vi "Add After Undo.vi"(11 "Test Case In":refnum<class "Undo Redo Core.lvclass">) -> (0 "error out":errorcluster, 3 "Test Case Out":refnum<class "Undo Redo Core.lvclass">)   [LabVIEW 2021, in "Undo Redo Core.lvclass"]
uses:
  Undo Redo Core.lvclass
  <resource>/plugins/NIIconEditor/Controls/Undo Redo Action.ctl
  4993e8ee-a06a-463a-9684-69129f64d5ce.vi
panel:
  out "Additional Add Variables":T1
  out "Undo Variables":T2(array[cluster])
  out "Current State Variables":T1
  out "Add Variables":T2(array[cluster])
  out "Undo State Output":string[](array[string])
  out "Current State":string
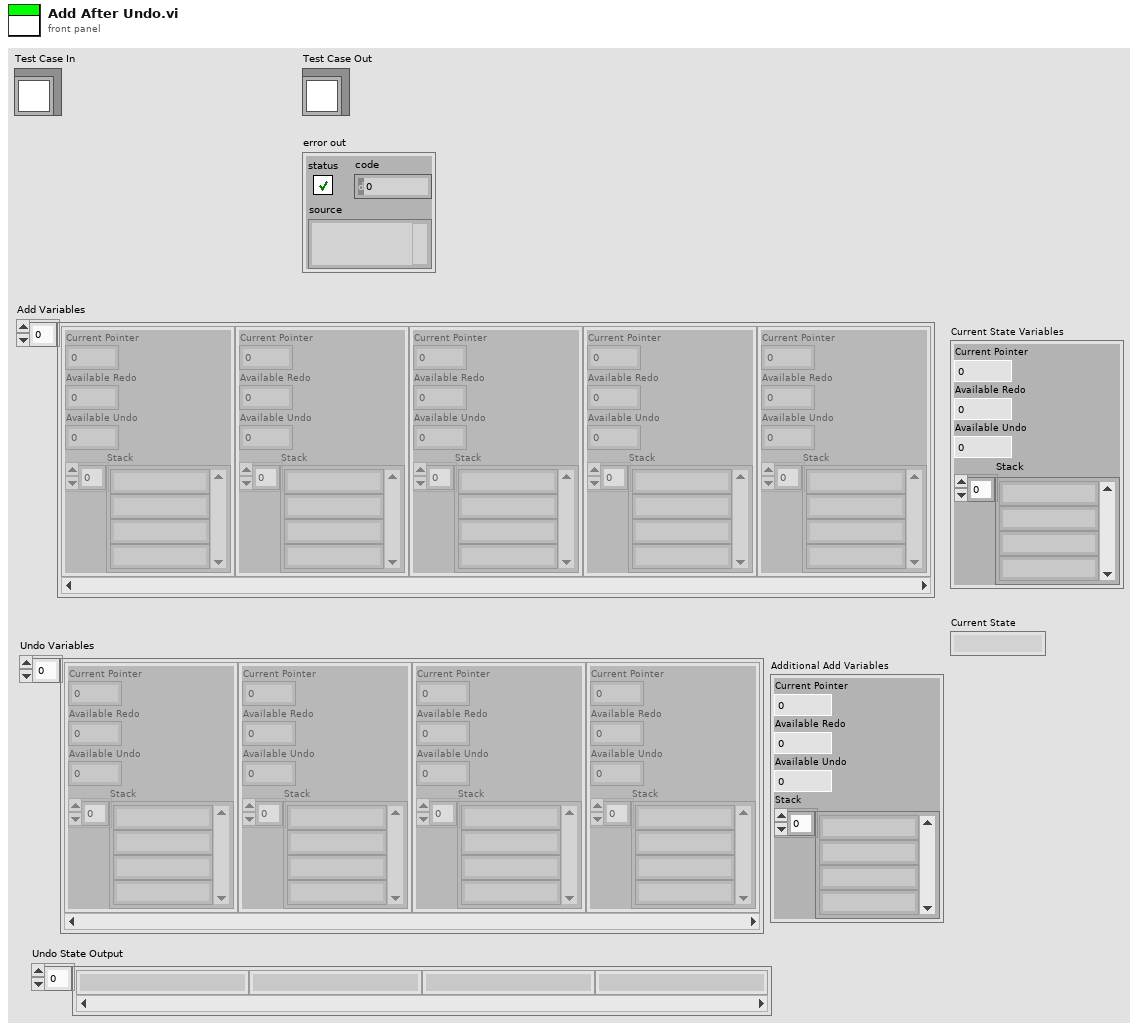
[diagram p1: front panel]
types:
  T1 = cluster{"Current Pointer":i32, "Available Redo":i32, "Available Undo":i32, "Stack":string[]}
  T2 = cluster{"Current Pointer":i32, "Available Redo":i32, "Available Undo":i32, "Stack":string[]}[]
  T3 = typedef "Undo Redo Action.ctl" = enum16{"Init", "Add", "Undo", "Redo", "Current State"}
  T4 = cluster{"Current Pointer":i32, "Available Redo":i32, "Available Undo":i32, "Buffer":string[]}
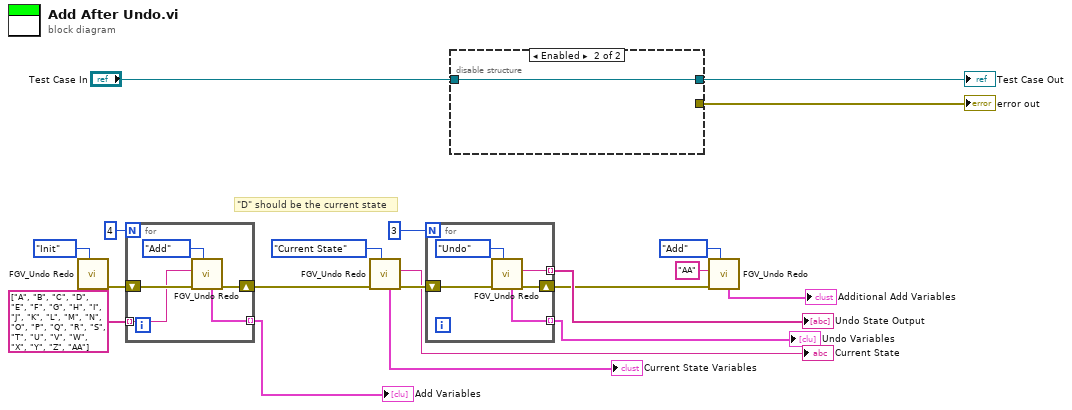
[diagram p0: block diagram]
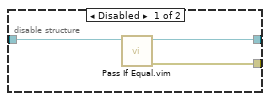
[diagram p2: hidden frame]
diagram:
  # "\"D\" should be the current state"
  n1 = call <resource>:"FGV_Undo Redo.vi"("Action"=Undo_Redo_Action."Init") -> ("error out"=w19:errorcluster)  [unwired: 8 in, 2 out]
  n2 = for {
    N: 4 -> [_]
    tunnel: string[] ["A", "B", "C", "D", "E", "F", "G", "H", "I", "J", "K", "L", "M", "N", "O", "P", "Q", "R", "S", "T", "U", "V", "W", "X", "Y", "Z", "AA"] -> [w22] mode=indexing
    shift-right: [w24] -> w18
    shift-left: w19 -> [w25]
    tunnel: [w21] -> w5 mode=indexing
    n3 = call <resource>:"FGV_Undo Redo.vi"("Action"=Undo_Redo_Action."Add", "error in"=w25, "State in"=w22) -> ("error out"=w24:errorcluster, "Internal Variables"=w21:T4)  [unwired: 6 in, 1 out]
  }
  "Add Variables" <- w5
  n4 = call <resource>:"FGV_Undo Redo.vi"("Action"=Undo_Redo_Action."Current State", "error in"=w18) -> ("error out"=w17:errorcluster, "State out"=→"Current State":string, "Internal Variables"=→"Current State Variables":T4)  [unwired: 7 in]
  n5 = for {
    N: 3 -> [_]
    shift-right: [w29] -> w7
    shift-left: w17 -> [w30]
    tunnel: [w27] -> w3 mode=indexing
    tunnel: [w26] -> w9 mode=indexing
    n6 = call <resource>:"FGV_Undo Redo.vi"("Action"=Undo_Redo_Action."Undo", "error in"=w30) -> ("error out"=w29:errorcluster, "State out"=w26:string, "Internal Variables"=w27:T4)  [unwired: 7 in]
  }
  "Undo State Output" <- w9
  "Undo Variables" <- w3
  n7 = disable-structure shown="Enabled" {
    disable-tunnel: "Test Case In" -> [w32 w34]
    disable-tunnel: [w31 w34] -> w15
    disable-tunnel: [w33 _] -> w20
    frame Disabled {
      n8 = call "Pass If Equal.vim"("LUnit Test Case In"=w32) -> ("error out"=w33:errorcluster, "LUnit Test Case Out"=w31:refnum<class "Undo Redo Core.lvclass">)  [unwired: 9 in]
    }
    frame Enabled {
    }
  }
  "error out" <- w20
  "Test Case Out" <- w15
  n9 = call <resource>:"FGV_Undo Redo.vi"("Action"=Undo_Redo_Action."Add", "error in"=w7, "State in"="AA" ("Data in")) -> ("Internal Variables"=→"Additional Add Variables":T4)  [unwired: 6 in, 2 out]
